vi "ShowGT_CrdStart.vi"(3 "fifo in":i16, 4 "crd in":i16, 5 "rtn_In":cluster{"rtn":i16, "Func":string}) -> (0 "fifo out":i16, 1 "crd out":i16, 2 "rtn_Out":cluster{"rtn":i16, "Func":string})   [LabVIEW 2014]
uses:
  VC6/gts.dll
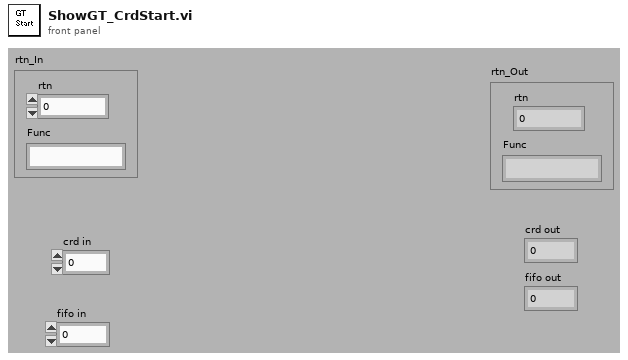
[diagram p1: front panel]
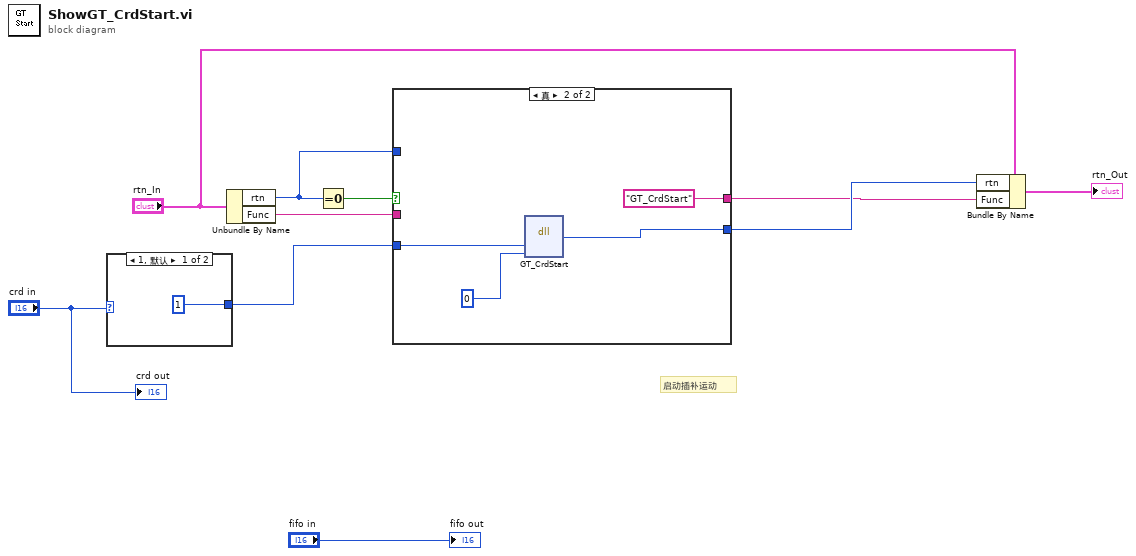
[diagram p0: block diagram]
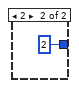
[diagram p2: hidden frame]
diagram:
  # "启动插补运动"
  n1 = case shown="1, 默认" "crd in" {
    tunnel: [i16 1 ("mask") i16 2 ("mask")] -> w2
    frame 1, Default {
    }
    frame 2 {
    }
  }
  n2 = Unbundle By Name("rtn_In") -> ("rtn"=w4:i16, "Func"=w5:string)
  n3 = Equal To 0?(x=w4) -> (x = 0?=w10:bool)
  n4 = case shown="真" w10 {
    tunnel: [w13 w18] -> w7
    tunnel: [w14 "GT_CrdStart" ("Func")] -> w6
    tunnel: w2 -> [_ w16]
    tunnel: w5 -> [w14 _]
    tunnel: w4 -> [w13 _]
    frame False {
    }
    frame True {
      n5 = dll-call lib="PTH2Fabs DNewGTS AC-800LWin7版源程序-20170926gts85VC6gts.dll" fn="GT_CrdStart"("mask"=w16, "option"=i16 0) -> ("rtn"=w18:i16)  [unwired: 5 in, 2 out]
    }
  }
  n6 = Bundle By Name(cluster="rtn_In", "rtn"=w7, "Func"=w6) -> (→"rtn_Out":cluster{"rtn":i16, "Func":string})
  "crd out" <- "crd in"
  "fifo out" <- "fifo in"
